vi "Get References to Controls in Front Panel Cluster.vi"(8 "error in (no error)":errorcluster, 10 "Items in Cluster":string[](array[string]), 11 "Clust Refnum":refnum<vi>) -> (0 "error out":errorcluster, 3 "References to Items":refnum<vi>[](array[refnum]))   [LabVIEW 2014]
panel:
  # "OR"
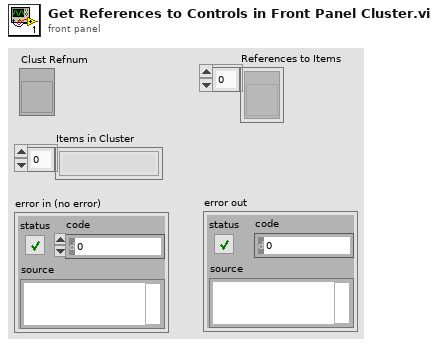
[diagram p1: front panel]
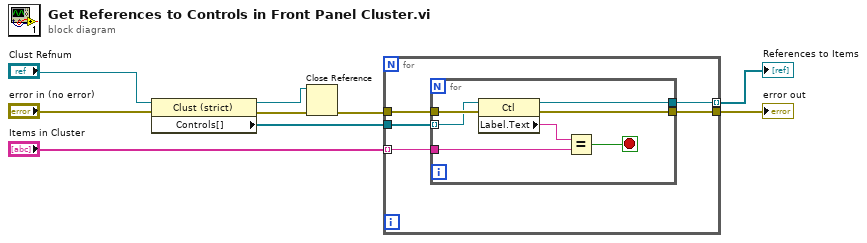
[diagram p0: block diagram]
diagram:
  n1 = property class="Clust (strict)"(reference="Clust Refnum", error in="error in (no error)") -> (reference out=w2:refnum<vi>, error out=w4:errorcluster, "Controls[]"=w7:refnum<vi>[])
  n2 = Close Reference(reference=w2, error in (no error)=w4) -> (error out=w3:errorcluster)
  n3 = for {
    tunnel: w3 -> [w14]
    tunnel: w7 -> [w13]
    tunnel: "Items in Cluster" -> [w12] mode=indexing
    tunnel: [w11] -> w9 mode=indexing
    tunnel: [w10] -> w5
    n4 = for {
      tunnel: w14 -> [w21]
      tunnel: w13 -> [w20] mode=indexing
      tunnel: w12 -> [w18]
      tunnel: [w17] -> w11
      tunnel: [w15] -> w10
      stop <- w16 stop-if-true
      n5 = property class="Ctl"(reference=w20, error in=w21) -> (reference out=w17:refnum<vi>, error out=w15:errorcluster, "Label.Text"=w19:string)
      n6 = Equal?(x=w19, y=w18) -> (x = y?=w16:bool)
    }
  }
  "References to Items" <- w9
  "error out" <- w5
